vi "SIAM-StackContinous.vi"(7 "Constants":T2={"Camera-StartLine"=1, "Camera-Endline"=1024, "Trigger_ticks"=10, "zAccel"=0.05, "z-delay-ticks"=700, "SCMOS-LineSpeed [10µs]"=2.7766} {"SCMOS-LineSpeed [10µs]" format="%#.6f" items=["Fast-285MHz"=0.9175, "Slow-95MHz"=2.7525, "Slow4.2"=2.7766]}, 8 "error in (no error)":errorcluster, 11 "User":T3={"z-distance_counts"=-500, "#planes"=20, "Digital-out"=enum."Laser0", "exposue [10µs]"=9600} {"#planes" min=1}) -> (0 "error out":errorcluster, 1 "SIAMScript":T5(array[cluster])=[{"Delay 10µs"=0, "command"=3489660929, "P0"=1048576, "P1"=1048576, "P2"=0, "P3"=0, "P4"=0, "P5-ticket"=0}, {"Delay 10µs"=10, "command"=3489660929, "P0"=1, "P1"=1, "P2"=0, "P3"=0, "P4"=0, "P5-ticket"=0}, {"Delay 10µs"=0, "command"=104857633, "P0"=-213, "P1"=0, "P2"=0, "P3"=0, "P4"=0, "P5-ticket"=0}, {"Delay 10µs"=192000, "command"=3489660929, "P0"=1, "P1"=0, "P2"=0, "P3"=0, "P4"=0, "P5-ticket"=0}, {"Delay 10µs"=0, "command"=104857633, "P0"=0, "P1"=0, "P2"=0, "P3"=0, "P4"=0, "P5-ticket"=0}, {"Delay 10µs"=2840, "command"=3489660929, "P0"=1048576, "P1"=0, "P2"=0, "P3"=0, "P4"=0, "P5-ticket"=0}, {"Delay 10µs"=50, "command"=104857729, "P0"=2560000, "P1"=0, "P2"=0, "P3"=0, "P4"=0, "P5-ticket"=0}, {"Delay 10µs"=10, "command"=4027518991, "P0"=0, "P1"=0, "P2"=0, "P3"=0, "P4"=0, "P5-ticket"=112}] {"command" format="%x" items=["read_x-Motor_status_ticket"=17305600, "init_x-Motor"=17760263, "read_x-Motor_absolute_ticket"=16781312, "move_x-Motor_absolute"=16777217, "move_x-Motor_relative"=16842753, "read_x-Motor_speed"=16977920, "set_x-Motor_speed"=16973825, "read_y-Motor_status_ticket"=18354176, "init_y-Motor"=18808839, "read_y-Motor_absolute_ticket"=17829888, "move_y-Motor_absolute"=17825793, "move_y-Motor_relative"=17891329, "read_y-Motor_speed"=18026496, "set_y-Motor_speed"=18022401, "read_z-Motor_status_ticket"=19402752, "init_z-Motor"=19857415, "stop_z-Motor"=19857423, "start_z-Motor"=19857422, "read_z-Motor_absolute_ticket"=18878464, "move_z-Motor_absolute"=18874369, "move_z-Motor_relative"=18939905, "read_Objective_status_ticket"=20451328, "init_Objective"=20905991, "read_Objective_absolute_ticket"=19927040, "move_Objective_absolute"=19922945, "move_Objective_relative"=19988481, "read_Objective-Motor_speed"=20123648, "set_Objective-Motor_speed"=20119553, "read_Filter_status_ticket"=21499904, "init_Filter"=21954567, "read_Filter_absolute_ticket"=20975616, "move_Filter_absolute"=20971521, "move_Filter_relative"=21037057, "read_Filter-Motor_speed"=21172224, "set_Filter-Motor_speed"=21168129, "read_Trans-Rad_status_ticket"=22548480, "init_Trans-Rad"=23003143, "read_Trans-Rad_absolute_ticket"=22024192, "move_Trans-Rad_absolute"=22020097, "move_Trans-Rad_relative"=22085633, "read_Trans-Motor_speed"=22220800, "set_Trans-Motor_speed"=22216705, "read_FRET_status_ticket"=23597056, "init_FRET"=24051719, "read_FRET_absolute_ticket"=23072768, "move_FRET_absolute"=23068673, "move_FRET_relative"=23134209, "read_FRET-Motor_speed"=23269376, "set_FRET-Motor_speed"=23265281, "read_SI-Rad_status_ticket"=24645632, "init_SI-Rad"=25100295, "read_SI-Rad_absolute_ticket"=24121344, "move_SI-Rad_absolute"=24117249, "move_SI-Rad_relative"=24182785, "read_SI-Rad_speed"=24317952, "set_SI-Rad_speed"=24313857, "I2C-write"=335544321, "I2C-read"=335548416, "end_no_ticket"=4027514895, "end_ticket"=4027518991, "IO-read_bank0"=3489665024, "IO-write_bank0"=3489660929, "IO-read_bank1"=3506442240, "IO-write_bank1"=3506438145, "DA0-0_LED365"=2684354561, "DA0-1_LED385"=2685403137, "DA0-2_LED440"=2686451713, "DA0-3_LED470"=2687500289, "DA0-4_LED510"=2688548865, "DA0-5_LED550"=2689597441, "DA0-6_LED590"=2690646017, "DA0-7_LED640"=2691694593, "DA1-0_LED-R"=2701131777, "DA1-1_LED-G"=2702180353, "DA1-2_LED-B"=2703228929, "DA1-3_LED-AF"=2704277505, "DA1-4"=2705326081, "DA1-5"=2706374657, "DA1-6"=2707423233, "DA1-7"=2708471809, "DA2-Laser0"=2717908993, "DA2-Laser1"=2718957569, "DA2-Laser2"=2720006145, "DA2-Laser3"=2721054721, "DA2-Laser4"=2722103297, "Analog-read_AD0-0"=2818576384, "Analog-read-store_AD0-0"=2818572290, "IO-delay_bank0"=3489923073, "IO-delay_bank0_fromVar"=3489923075, "read_cam_clock"=3289124864, "store_cam_clock"=3289120770, "read_cam_phase"=3289190400, "store_cam_phase"=3289190402, "Read ticks"=4027518976, "Read ticks to var"=4027518978, "Read IP"=4043313152, "Read IP into var"=4043313154, "Set IP from var"=4043309059, "Set IP from var, relative"=4043313155, "decrement_branchRel_if_equal"=4043374945, "decrement_branchRel_if_greaterequal"=4043375201, "decrement_branchRel_if_greaterequal_withTicket"=4043379297, "decrement_branchRel_if_smaller"=4043375457, "increment_branchRel_if_smaller"=4043375473, "readVar"=4060090368, "writeVar"=4060086273, "readVar_and_copy_to_var2"=4060086275, "loadVar2_andcopy_var1"=4060086276, "math_addToVariable"=4076863488, "math_addVToVariable"=4076863489, "math_subToVariable"=4076863490, "math_subVToVariable"=4076863491, "math_multToVariable"=4076863492, "math_multvToVariable"=4076863493, "math_divideToVariable"=4076863494, "math_divideVToVariable"=4076863495, "math_modToVariable"=4076863496, "math_modVToVariable"=4076863497, "logic_and"=4093640704, "logic_or"=4093640706, "logic_xor"=4093640708, "set_1Galvo"=101712113, "set_x-Galvo"=102760689, "set_y-Galvo"=103809265, "set_z-Fokus"=104857841, "set_1Galvo_position-only"=101711937, "set_x-Galvo_position-only"=102760513, "set_y-Galvo_position-only"=103809089, "set_z-Fokus_position-only"=104857665, "set_x-Galvo_position-only_ticket"=102764609, "set_y-Galvo_position-only_ticket"=103813185, "set_z-Fokus_position-only_ticket"=104861761, "set_x-Galvo_relativ-only"=102760577, "set_y-Galvo_relativ-only"=103809153, "set_z-Fokus_relativ-only"=104857729, "set_x-Galvo_speed-only"=102760481, "set_y-Galvo_speed-only"=103809057, "set_z-Fokus_speed-only"=104857633, "read_1Galvo_ticket"=101716032, "read_x-Galvo_ticket"=102764608, "read_y-Galvo_ticket"=103813184, "read_z-Focus_ticket"=104861760, "x-Galvo_pos_fromVar"=102760515, "y-Galvo_pos_fromVar"=103809091, "z-Focus_pos_fromVar"=104857667, "Servo0"=67108865, "Servo0-enable"=68091911, "Servo0-disable"=68091919, "Servo1"=68157441, "Servo1-enable"=69140487, "Servo1-disable"=69140495, "EnablePower0-SM"=2148466695, "DisablePower0-SM"=2148466703, "EnablePower1-Thermo1"=2149515271, "DisablePower1-Thermo1"=2149515279, "EnablePower2-Cam"=2150563847, "DisablePower2-Cam"=2150563855, "EnablePower3-Thermo2"=2151612423, "DisablePower3-Thermo2"=2151612431, "EnablePower4-Laser0"=2152660999, "DisablePower4-Laser0"=2152661007, "EnablePower5"=2153709575, "DisablePower5"=2153709583, "EnablePower6-Laser1"=2154758151, "DisablePower6-Laser1"=2154758159, "EnablePower7-SAM"=2155806727, "DisablePower7-SAM"=2155806735, "EnablePower8-Laser2"=2156855303, "DisablePower8-Laser2"=2156855311, "EnablePower9-TSM"=2157903879, "DisablePower9-TSM"=2157903887, "EnablePower10-Laser3"=2158952455, "DisablePower10-Laser3"=2158952463, "EnablePower11-Servo"=2160001031, "DisablePower11-Servo"=2160001039, "EnablePower12-Laser4"=2161049607, "DisablePower12-Laser4"=2161049615, "EnableSMPower2-DCC22"=2167341063, "DisableSMPower2-DCC22"=2167341071, "EnableSMPower3-6220"=2168389639, "DisableSMPower3-6220"=2168389647, "EnableSMPower4-6210"=2169438215, "DisableSMPower4-6210"=2169438223]}, 2 "Camera":T1={"Camera-Exposure µs"=96000.0, "CameraImages"=20})   [LabVIEW 2011]
uses:
  SIAM_command.ctl
panel:
  out "readout":u32=2840
  out "size(s)":i32=8
  # "1.laser an\n2. trigger an\n3. linaer z bewegen, linear geht naicht also lauter schritte\n4. trigger aus\n5. laser aus\n6. z stop, Readout später!\n7. z zurück\n8 ende\nCamware macht sequenz!"
  # "var0=phase\nvar1=clock256\nvar 2 =linecounter \nvar 3 =framecounter"
  # "<-- user inputs --------------------------- constants ---->"
  # "-250 count = 500nm"
  # "Pixel definition: 0\nmiddel: lines\nbottom +2lines"
  # "alles umstellen auf count und Pixel und 10µs !!!"
  # "lineclock read slow=AD99E =711070 =/256=27.77617"
  # "a gerechnet wobbler~3.7, x~98, eher /2\nz~6ms/2µm"
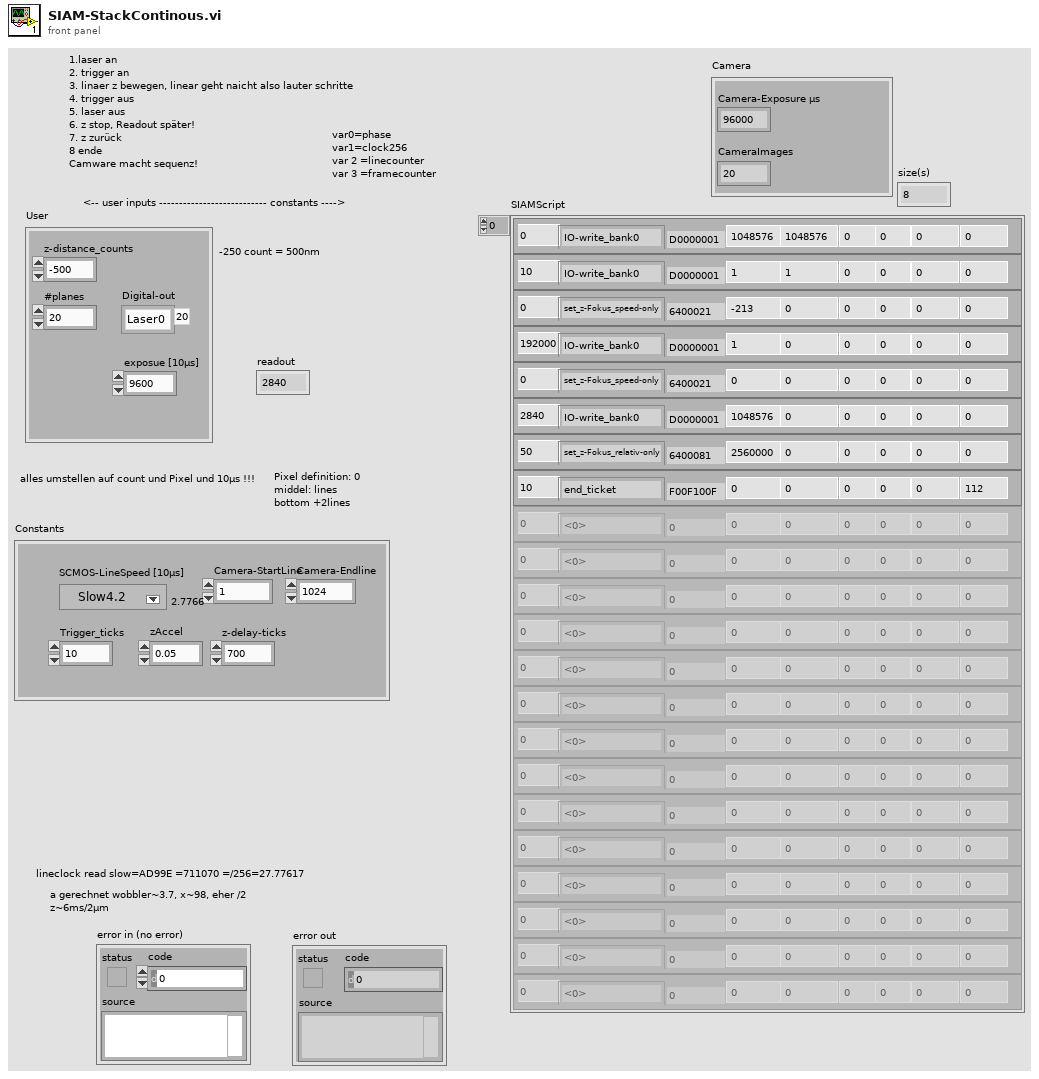
[diagram p1: front panel]
types:
  T1 = cluster{"Camera-Exposure µs":dbl, "CameraImages":u16}
  T2 = cluster{"Camera-StartLine":u32, "Camera-Endline":u32, "Trigger_ticks":u32, "zAccel":dbl, "z-delay-ticks":u32, "SCMOS-LineSpeed [10µs]":dbl}
  T3 = cluster{"z-distance_counts":i32, "#planes":u16, "Digital-out":enum8{"cam1", "cam1-ready?", "cam2", "cam2-ready?", "tmsx?", "tsmy?", "tsm3?", "lid?", "led1", "led2", "led3", "led4", "led5", "led6", "led7", "led8", "durchR", "durchG", "durchB", "AF", "Laser0", "Laser1", "Laser2", "Laser3", "Laser4", "LaserX", "TrigOut", "SMB1", ""}, "exposue [10µs]":u32}
  T4 = typedef "SIAM_command.ctl" = u32
  T5 = cluster{"Delay 10µs":u32, "command":T4, "P0":i32, "P1":i32, "P2":i32, "P3":i32, "P4":i32, "P5-ticket":i32}[]
  T6 = cluster{"Delay 10µs":u32, "command":T4, "P0":i32, "P1":i32, "P2":i32, "P3":i32, "P4":i32, "P5-ticket":i32}
  T7 = cluster{"Camera-Exposure":dbl, "CameraImages":u16}
  T8 = enum8{"Ch0", "Ch1", "x-Galvo", "y-Galvo", "z-Focus"}
  T9 = enum8{"cam1", "cam1-ready?", "cam2", "cam2-ready?", "tmsx?", "tsmy?", "tsm3?", "lid?", "led1", "led2", "led3", "led4", "led5", "led6", "led7", "led8", "durchR", "durchG", "durchB", "AF", "Laser0", "Laser1", "Laser2", "Laser3", "Laser4", "LaserX", "TrigOut", "SMB1", ""}
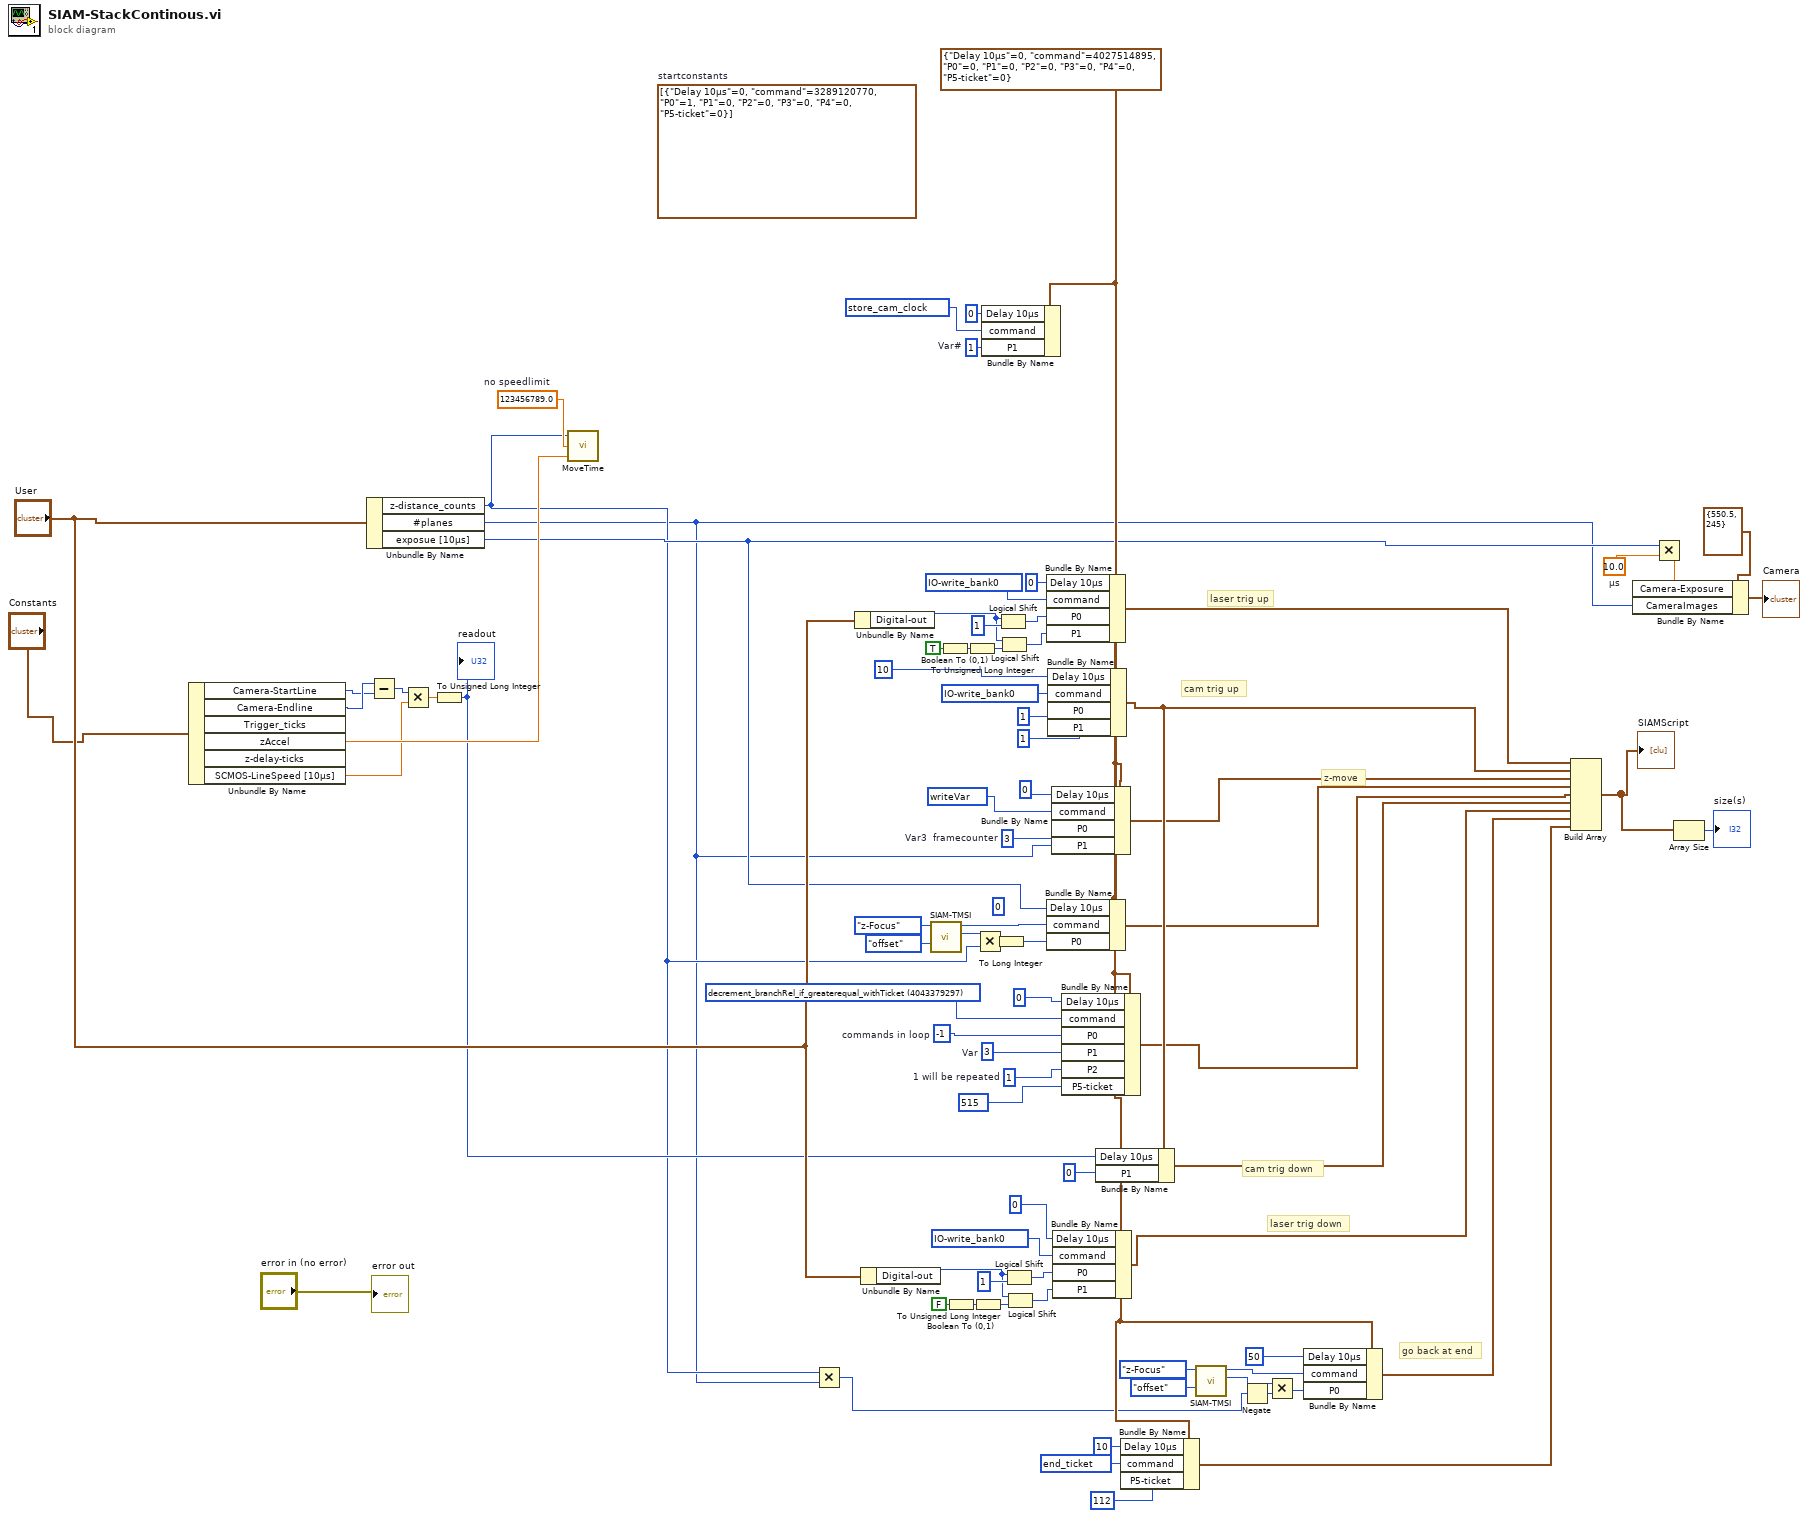
[diagram p0: block diagram]
diagram:
  w11 = 1  # 1 will be repeated
  w13 = 3  # Var
  w10 = -1  # commands in loop
  w14 = T4 4043379297 items=["read_x-Motor_status_ticket"=17305600, "init_x-Motor"=17760263, "read_x-Motor_absolute_ticket"=16781312, "move_x-Motor_absolute"=16777217, "move_x-Motor_relative"=16842753, "read_x-Motor_speed"=16977920, "set_x-Motor_speed"=16973825, "read_y-Motor_status_ticket"=18354176, "init_y-Motor"=18808839, "read_y-Motor_absolute_ticket"=17829888, "move_y-Motor_absolute"=17825793, "move_y-Motor_relative"=17891329, "read_y-Motor_speed"=18026496, "set_y-Motor_speed"=18022401, "read_z-Motor_status_ticket"=19402752, "init_z-Motor"=19857415, "stop_z-Motor"=19857423, "start_z-Motor"=19857422, "read_z-Motor_absolute_ticket"=18878464, "move_z-Motor_absolute"=18874369, "move_z-Motor_relative"=18939905, "read_Objective_status_ticket"=20451328, "init_Objective"=20905991, "read_Objective_absolute_ticket"=19927040, "move_Objective_absolute"=19922945, "move_Objective_relative"=19988481, "read_Objective-Motor_speed"=20123648, "set_Objective-Motor_speed"=20119553, "read_Filter_status_ticket"=21499904, "init_Filter"=21954567, "read_Filter_absolute_ticket"=20975616, "move_Filter_absolute"=20971521, "move_Filter_relative"=21037057, "read_Filter-Motor_speed"=21172224, "set_Filter-Motor_speed"=21168129, "read_Trans-Rad_status_ticket"=22548480, "init_Trans-Rad"=23003143, "read_Trans-Rad_absolute_ticket"=22024192, "move_Trans-Rad_absolute"=22020097, "move_Trans-Rad_relative"=22085633, "read_Trans-Motor_speed"=22220800, "set_Trans-Motor_speed"=22216705, "read_FRET_status_ticket"=23597056, "init_FRET"=24051719, "read_FRET_absolute_ticket"=23072768, "move_FRET_absolute"=23068673, "move_FRET_relative"=23134209, "read_FRET-Motor_speed"=23269376, "set_FRET-Motor_speed"=23265281, "read_SI-Rad_status_ticket"=24645632, "init_SI-Rad"=25100295, "read_SI-Rad_absolute_ticket"=24121344, "move_SI-Rad_absolute"=24117249, "move_SI-Rad_relative"=24182785, "read_SI-Rad_speed"=24317952, "set_SI-Rad_speed"=24313857, "end_no_ticket"=4027514895, "end_ticket"=4027518991, "IO-read_bank0"=3489665024, "IO-write_bank0"=3489660929, "IO-read_bank1"=3506442240, "IO-write_bank1"=3506438145, "DA0-0_LED365"=2684354561, "DA0-1_LED385"=2685403137, "DA0-2_LED440"=2686451713, "DA0-3_LED470"=2687500289, "DA0-4_LED510"=2688548865, "DA0-5_LED550"=2689597441, "DA0-6_LED590"=2690646017, "DA0-7_LED640"=2691694593, "DA1-0_LED-R"=2701131777, "DA1-1_LED-G"=2702180353, "DA1-2_LED-B"=2703228929, "DA1-3_LED-AF"=2704277505, "DA1-4"=2705326081, "DA1-5"=2706374657, "DA1-6"=2707423233, "DA1-7"=2708471809, "DA2-Laser0"=2717908993, "DA2-Laser1"=2718957569, "DA2-Laser2"=2720006145, "DA2-Laser3"=2721054721, "DA2-Laser4"=2722103297, "Analog-read_AD0-0"=2818576384, "Analog-read-store_AD0-0"=2818572290, "IO-delay_bank0"=3489923073, "IO-delay_bank0_fromVar"=3489923075, "read_cam_clock"=3289124864, "store_cam_clock"=3289120770, "read_cam_phase"=3289190400, "store_cam_phase"=3289190402, "Read ticks"=4027518976, "Read ticks to var"=4027518978, "Read IP"=4043313152, "Read IP into var"=4043313154, "Set IP from var"=4043309059, "Set IP from var, relative"=4043313155, "decrement_branchRel_if_equal"=4043374945, "decrement_branchRel_if_greaterequal"=4043375201, "decrement_branchRel_if_greaterequal_withTicket"=4043379297, "decrement_branchRel_if_smaller"=4043375457, "increment_branchRel_if_smaller"=4043375473, "readVar"=4060090368, "writeVar"=4060086273, "readVar_and_copy_to_var2"=4060086275, "loadVar2_andcopy_var1"=4060086276, "math_addToVariable"=4076863488, "math_addVToVariable"=4076863489, "math_subToVariable"=4076863490, "math_subVToVariable"=4076863491, "math_multToVariable"=4076863492, "math_multvToVariable"=4076863493, "math_divideToVariable"=4076863494, "math_divideVToVariable"=4076863495, "math_modToVariable"=4076863496, "math_modVToVariable"=4076863497, "logic_and"=4093640704, "logic_or"=4093640706, "logic_xor"=4093640708, "set_1Galvo"=101712113, "set_x-Galvo"=102760689, "set_y-Galvo"=103809265, "set_z-Fokus"=104857841, "set_1Galvo_position-only"=101711937, "set_x-Galvo_position-only"=102760513, "set_y-Galvo_position-only"=103809089, "set_z-Fokus_position-only"=104857665, "set_x-Galvo_position-only_ticket"=102764609, "set_y-Galvo_position-only_ticket"=103813185, "set_z-Fokus_position-only_ticket"=104861761, "set_x-Galvo_relativ-only"=102760577, "set_y-Galvo_relativ-only"=103809153, "set_z-Fokus_relativ-only"=104857729, "set_x-Galvo_speed-only"=102760481, "set_y-Galvo_speed-only"=103809057, "set_z-Fokus_speed-only"=104857633, "read_1Galvo_ticket"=101716032, "read_x-Galvo_ticket"=102764608, "read_y-Galvo_ticket"=103813184, "read_z-Focus_ticket"=104861760, "x-Galvo_pos_fromVar"=102760515, "y-Galvo_pos_fromVar"=103809091, "z-Focus_pos_fromVar"=104857667, "Servo0"=67108865, "Servo0-enable"=68091911, "Servo0-disable"=68091919, "Servo1"=68157441, "Servo1-enable"=69140487, "Servo1-disable"=69140495, "EnablePower0-SM"=2148466695, "DisablePower0-SM"=2148466703, "EnablePower1-Thermo1"=2149515271, "DisablePower1-Thermo1"=2149515279, "EnablePower2-Cam"=2150563847, "DisablePower2-Cam"=2150563855, "EnablePower3-Thermo2"=2151612423, "DisablePower3-Thermo2"=2151612431, "EnablePower4-Laser0"=2152660999, "DisablePower4-Laser0"=2152661007, "EnablePower5"=2153709575, "DisablePower5"=2153709583, "EnablePower6-Laser1"=2154758151, "DisablePower6-Laser1"=2154758159, "EnablePower7-SAM"=2155806727, "DisablePower7-SAM"=2155806735, "EnablePower8-Laser2"=2156855303, "DisablePower8-Laser2"=2156855311, "EnablePower9-TSM"=2157903879, "DisablePower9-TSM"=2157903887, "EnablePower10-Laser3"=2158952455, "DisablePower10-Laser3"=2158952463, "EnablePower11-Servo"=2160001031, "DisablePower11-Servo"=2160001039, "EnablePower12-Laser4"=2161049607, "DisablePower12-Laser4"=2161049615, "EnableSMPower2-DCC22"=2167341063, "DisableSMPower2-DCC22"=2167341071, "EnableSMPower3-6220"=2168389639, "DisableSMPower3-6220"=2168389647, "EnableSMPower4-6210"=2169438215, "DisableSMPower4-6210"=2169438223] ("command")
  w15 = 3  # Var3  framecounter
  w17 = T4 4060086273 items=["read_x-Motor_status_ticket"=17305600, "init_x-Motor"=17760263, "read_x-Motor_absolute_ticket"=16781312, "move_x-Motor_absolute"=16777217, "move_x-Motor_relative"=16842753, "read_x-Motor_speed"=16977920, "set_x-Motor_speed"=16973825, "read_y-Motor_status_ticket"=18354176, "init_y-Motor"=18808839, "read_y-Motor_absolute_ticket"=17829888, "move_y-Motor_absolute"=17825793, "move_y-Motor_relative"=17891329, "read_y-Motor_speed"=18026496, "set_y-Motor_speed"=18022401, "read_z-Motor_status_ticket"=19402752, "init_z-Motor"=19857415, "stop_z-Motor"=19857423, "start_z-Motor"=19857422, "read_z-Motor_absolute_ticket"=18878464, "move_z-Motor_absolute"=18874369, "move_z-Motor_relative"=18939905, "read_Objective_status_ticket"=20451328, "init_Objective"=20905991, "read_Objective_absolute_ticket"=19927040, "move_Objective_absolute"=19922945, "move_Objective_relative"=19988481, "read_Objective-Motor_speed"=20123648, "set_Objective-Motor_speed"=20119553, "read_Filter_status_ticket"=21499904, "init_Filter"=21954567, "read_Filter_absolute_ticket"=20975616, "move_Filter_absolute"=20971521, "move_Filter_relative"=21037057, "read_Filter-Motor_speed"=21172224, "set_Filter-Motor_speed"=21168129, "read_Trans-Rad_status_ticket"=22548480, "init_Trans-Rad"=23003143, "read_Trans-Rad_absolute_ticket"=22024192, "move_Trans-Rad_absolute"=22020097, "move_Trans-Rad_relative"=22085633, "read_Trans-Motor_speed"=22220800, "set_Trans-Motor_speed"=22216705, "read_FRET_status_ticket"=23597056, "init_FRET"=24051719, "read_FRET_absolute_ticket"=23072768, "move_FRET_absolute"=23068673, "move_FRET_relative"=23134209, "read_FRET-Motor_speed"=23269376, "set_FRET-Motor_speed"=23265281, "read_SI-Rad_status_ticket"=24645632, "init_SI-Rad"=25100295, "read_SI-Rad_absolute_ticket"=24121344, "move_SI-Rad_absolute"=24117249, "move_SI-Rad_relative"=24182785, "read_SI-Rad_speed"=24317952, "set_SI-Rad_speed"=24313857, "end_no_ticket"=4027514895, "end_ticket"=4027518991, "IO-read_bank0"=3489665024, "IO-write_bank0"=3489660929, "IO-read_bank1"=3506442240, "IO-write_bank1"=3506438145, "DA0-0_LED365"=2684354561, "DA0-1_LED385"=2685403137, "DA0-2_LED440"=2686451713, "DA0-3_LED470"=2687500289, "DA0-4_LED510"=2688548865, "DA0-5_LED550"=2689597441, "DA0-6_LED590"=2690646017, "DA0-7_LED640"=2691694593, "DA1-0_LED-R"=2701131777, "DA1-1_LED-G"=2702180353, "DA1-2_LED-B"=2703228929, "DA1-3_LED-AF"=2704277505, "DA1-4"=2705326081, "DA1-5"=2706374657, "DA1-6"=2707423233, "DA1-7"=2708471809, "DA2-Laser0"=2717908993, "DA2-Laser1"=2718957569, "DA2-Laser2"=2720006145, "DA2-Laser3"=2721054721, "DA2-Laser4"=2722103297, "Analog-read_AD0-0"=2818576384, "Analog-read-store_AD0-0"=2818572290, "IO-delay_bank0"=3489923073, "IO-delay_bank0_fromVar"=3489923075, "read_cam_clock"=3289124864, "store_cam_clock"=3289120770, "read_cam_phase"=3289190400, "store_cam_phase"=3289190402, "Read ticks"=4027518976, "Read ticks to var"=4027518978, "Read IP"=4043313152, "Read IP into var"=4043313154, "Set IP from var"=4043309059, "Set IP from var, relative"=4043313155, "decrement_branchRel_if_equal"=4043374945, "decrement_branchRel_if_greaterequal"=4043375201, "decrement_branchRel_if_greaterequal_withTicket"=4043379297, "decrement_branchRel_if_smaller"=4043375457, "increment_branchRel_if_smaller"=4043375473, "readVar"=4060090368, "writeVar"=4060086273, "readVar_and_copy_to_var2"=4060086275, "loadVar2_andcopy_var1"=4060086276, "math_addToVariable"=4076863488, "math_addVToVariable"=4076863489, "math_subToVariable"=4076863490, "math_subVToVariable"=4076863491, "math_multToVariable"=4076863492, "math_multvToVariable"=4076863493, "math_divideToVariable"=4076863494, "math_divideVToVariable"=4076863495, "math_modToVariable"=4076863496, "math_modVToVariable"=4076863497, "logic_and"=4093640704, "logic_or"=4093640706, "logic_xor"=4093640708, "set_1Galvo"=101712113, "set_x-Galvo"=102760689, "set_y-Galvo"=103809265, "set_z-Fokus"=104857841, "set_1Galvo_position-only"=101711937, "set_x-Galvo_position-only"=102760513, "set_y-Galvo_position-only"=103809089, "set_z-Fokus_position-only"=104857665, "set_x-Galvo_position-only_ticket"=102764609, "set_y-Galvo_position-only_ticket"=103813185, "set_z-Fokus_position-only_ticket"=104861761, "set_x-Galvo_relativ-only"=102760577, "set_y-Galvo_relativ-only"=103809153, "set_z-Fokus_relativ-only"=104857729, "set_x-Galvo_speed-only"=102760481, "set_y-Galvo_speed-only"=103809057, "set_z-Fokus_speed-only"=104857633, "read_1Galvo_ticket"=101716032, "read_x-Galvo_ticket"=102764608, "read_y-Galvo_ticket"=103813184, "read_z-Focus_ticket"=104861760, "x-Galvo_pos_fromVar"=102760515, "y-Galvo_pos_fromVar"=103809091, "z-Focus_pos_fromVar"=104857667, "Servo0"=67108865, "Servo0-enable"=68091911, "Servo0-disable"=68091919, "Servo1"=68157441, "Servo1-enable"=69140487, "Servo1-disable"=69140495, "EnablePower0-SM"=2148466695, "DisablePower0-SM"=2148466703, "EnablePower1-Thermo1"=2149515271, "DisablePower1-Thermo1"=2149515279, "EnablePower2-Cam"=2150563847, "DisablePower2-Cam"=2150563855, "EnablePower3-Thermo2"=2151612423, "DisablePower3-Thermo2"=2151612431, "EnablePower4-Laser0"=2152660999, "DisablePower4-Laser0"=2152661007, "EnablePower5"=2153709575, "DisablePower5"=2153709583, "EnablePower6-Laser1"=2154758151, "DisablePower6-Laser1"=2154758159, "EnablePower7-SAM"=2155806727, "DisablePower7-SAM"=2155806735, "EnablePower8-Laser2"=2156855303, "DisablePower8-Laser2"=2156855311, "EnablePower9-TSM"=2157903879, "DisablePower9-TSM"=2157903887, "EnablePower10-Laser3"=2158952455, "DisablePower10-Laser3"=2158952463, "EnablePower11-Servo"=2160001031, "DisablePower11-Servo"=2160001039, "EnablePower12-Laser4"=2161049607, "DisablePower12-Laser4"=2161049615, "EnableSMPower2-DCC22"=2167341063, "DisableSMPower2-DCC22"=2167341071, "EnableSMPower3-6220"=2168389639, "DisableSMPower3-6220"=2168389647, "EnableSMPower4-6210"=2169438215, "DisableSMPower4-6210"=2169438223] ("command")
  w35 = 123456789.0  # no speedlimit
  w44 = T4 3489660929 items=["read_x-Motor_status_ticket"=17305600, "init_x-Motor"=17760263, "read_x-Motor_absolute_ticket"=16781312, "move_x-Motor_absolute"=16777217, "move_x-Motor_relative"=16842753, "read_y-Motor_status_ticket"=18354176, "init_y-Motor"=18808839, "read_y-Motor_absolute_ticket"=17829888, "move_y-Motor_absolute"=17825793, "move_y-Motor_relative"=17891329, "read_z-Motor_status_ticket"=19402752, "init_z-Motor"=19857415, "stop_z-Motor"=19857423, "start_z-Motor"=19857422, "read_z-Motor_absolute_ticket"=18878464, "move_z-Motor_absolute"=18874369, "move_z-Motor_relative"=18939905, "end_no_ticket"=4027514895, "end_ticket"=4027518991, "IO-read_bank0"=3489665024, "IO-write_bank0"=3489660929, "IO-read_bank1"=3506442240, "IO-write_bank1"=3506438145, "IO-delay_bank0"=3489923073, "IO-delay_bank0_fromVar"=3489923075, "read_cam_clock"=3289124864, "store_cam_clock"=3289120770, "read_cam_phase"=3289190400, "set_cam_deadtime"=3288989697, "set_cam_10uscycles"=3289055233, "set_cam_10uscycles_fromVariable"=3289055235, "calc_cam"=3289317386, "store_cam_Var"=3289251842, "math_addToVariable"=4060086278, "readVar"=4060090368, "writeVar"=4060086273, "copyVar"=4060086276, "decrement_branchRel_if_equal"=4043374945, "decrement_branchRel_if_greaterequal"=4043375201, "decrement_branchRel_if_greaterequal_withTicket"=4043379297, "decrement_branchRel_if_smaller"=4043375457, "increment_branchRel_if_smaller"=4043375473, "set_x-Galvo"=1612710129, "set_y-Galvo"=1613758705, "set_z-Fokus"=1614807281, "set_x-Galvo_position-only"=1612709953, "set_y-Galvo_position-only"=1613758529, "set_z-Fokus_position-only"=1614807105, "set_x-Galvo_position-only_ticket"=1612714049, "set_y-Galvo_position-only_ticket"=1613762625, "set_z-Fokus_position-only_ticket"=1614811201, "read_x-Galvo_ticket"=1612714048, "read_y-Galvo_ticket"=1613762624, "read_z-Focus_ticket"=1614811200, "x-Galvo_pos_fromVar"=1612709955, "y-Galvo_pos_fromVar"=1613758531, "z-Focus_pos_fromVar"=1614807107] ("command")
  w52 = T4 3489660929 items=["read_x-Motor_status_ticket"=17305600, "init_x-Motor"=17760263, "read_x-Motor_absolute_ticket"=16781312, "move_x-Motor_absolute"=16777217, "move_x-Motor_relative"=16842753, "read_y-Motor_status_ticket"=18354176, "init_y-Motor"=18808839, "read_y-Motor_absolute_ticket"=17829888, "move_y-Motor_absolute"=17825793, "move_y-Motor_relative"=17891329, "read_z-Motor_status_ticket"=19402752, "init_z-Motor"=19857415, "stop_z-Motor"=19857423, "start_z-Motor"=19857422, "read_z-Motor_absolute_ticket"=18878464, "move_z-Motor_absolute"=18874369, "move_z-Motor_relative"=18939905, "end_no_ticket"=4027514895, "end_ticket"=4027518991, "IO-read_bank0"=3489665024, "IO-write_bank0"=3489660929, "IO-read_bank1"=3506442240, "IO-write_bank1"=3506438145, "IO-delay_bank0"=3489923073, "IO-delay_bank0_fromVar"=3489923075, "read_cam_clock"=3289124864, "store_cam_clock"=3289120770, "read_cam_phase"=3289190400, "set_cam_deadtime"=3288989697, "set_cam_10uscycles"=3289055233, "set_cam_10uscycles_fromVariable"=3289055235, "calc_cam"=3289317386, "store_cam_Var"=3289251842, "math_addToVariable"=4060086278, "readVar"=4060090368, "writeVar"=4060086273, "copyVar"=4060086276, "decrement_branchRel_if_equal"=4043374945, "decrement_branchRel_if_greaterequal"=4043375201, "decrement_branchRel_if_greaterequal_withTicket"=4043379297, "decrement_branchRel_if_smaller"=4043375457, "increment_branchRel_if_smaller"=4043375473, "set_x-Galvo"=1612710129, "set_y-Galvo"=1613758705, "set_z-Fokus"=1614807281, "set_x-Galvo_position-only"=1612709953, "set_y-Galvo_position-only"=1613758529, "set_z-Fokus_position-only"=1614807105, "set_x-Galvo_position-only_ticket"=1612714049, "set_y-Galvo_position-only_ticket"=1613762625, "set_z-Fokus_position-only_ticket"=1614811201, "read_x-Galvo_ticket"=1612714048, "read_y-Galvo_ticket"=1613762624, "read_z-Focus_ticket"=1614811200, "x-Galvo_pos_fromVar"=1612709955, "y-Galvo_pos_fromVar"=1613758531, "z-Focus_pos_fromVar"=1614807107] ("command")
  w9 = T6 {"Delay 10µs"=0, "command"=4027514895, "P0"=0, "P1"=0, "P2"=0, "P3"=0, "P4"=0, "P5-ticket"=0} ("Cluster")
  (unwired) T5 [{"Delay 10µs"=0, "command"=3289120770, "P0"=1, "P1"=0, "P2"=0, "P3"=0, "P4"=0, "P5-ticket"=0}]  # startconstants
  w53 = 1  # Var#
  w54 = T4 3289120770 items=["read_x-Motor_status_ticket"=17305600, "init_x-Motor"=17760263, "read_x-Motor_absolute_ticket"=16781312, "move_x-Motor_absolute"=16777217, "move_x-Motor_relative"=16842753, "read_x-Motor_speed"=16977920, "set_x-Motor_speed"=16973825, "read_y-Motor_status_ticket"=18354176, "init_y-Motor"=18808839, "read_y-Motor_absolute_ticket"=17829888, "move_y-Motor_absolute"=17825793, "move_y-Motor_relative"=17891329, "read_y-Motor_speed"=18026496, "set_y-Motor_speed"=18022401, "read_z-Motor_status_ticket"=19402752, "init_z-Motor"=19857415, "stop_z-Motor"=19857423, "start_z-Motor"=19857422, "read_z-Motor_absolute_ticket"=18878464, "move_z-Motor_absolute"=18874369, "move_z-Motor_relative"=18939905, "read_Objective_status_ticket"=20451328, "init_Objective"=20905991, "read_Objective_absolute_ticket"=19927040, "move_Objective_absolute"=19922945, "move_Objective_relative"=19988481, "read_Objective-Motor_speed"=20123648, "set_Objective-Motor_speed"=20119553, "read_Filter_status_ticket"=21499904, "init_Filter"=21954567, "read_Filter_absolute_ticket"=20975616, "move_Filter_absolute"=20971521, "move_Filter_relative"=21037057, "read_Filter-Motor_speed"=21172224, "set_Filter-Motor_speed"=21168129, "read_Trans-Rad_status_ticket"=22548480, "init_Trans-Rad"=23003143, "read_Trans-Rad_absolute_ticket"=22024192, "move_Trans-Rad_absolute"=22020097, "move_Trans-Rad_relative"=22085633, "read_Trans-Motor_speed"=22220800, "set_Trans-Motor_speed"=22216705, "read_FRET_status_ticket"=23597056, "init_FRET"=24051719, "read_FRET_absolute_ticket"=23072768, "move_FRET_absolute"=23068673, "move_FRET_relative"=23134209, "read_FRET-Motor_speed"=23269376, "set_FRET-Motor_speed"=23265281, "read_SI-Rad_status_ticket"=24645632, "init_SI-Rad"=25100295, "read_SI-Rad_absolute_ticket"=24121344, "move_SI-Rad_absolute"=24117249, "move_SI-Rad_relative"=24182785, "read_SI-Rad_speed"=24317952, "set_SI-Rad_speed"=24313857, "I2C-write"=335544321, "I2C-read"=335548416, "end_no_ticket"=4027514895, "end_ticket"=4027518991, "IO-read_bank0"=3489665024, "IO-write_bank0"=3489660929, "IO-read_bank1"=3506442240, "IO-write_bank1"=3506438145, "DA0-0_LED365"=2684354561, "DA0-1_LED385"=2685403137, "DA0-2_LED440"=2686451713, "DA0-3_LED470"=2687500289, "DA0-4_LED510"=2688548865, "DA0-5_LED550"=2689597441, "DA0-6_LED590"=2690646017, "DA0-7_LED640"=2691694593, "DA1-0_LED-R"=2701131777, "DA1-1_LED-G"=2702180353, "DA1-2_LED-B"=2703228929, "DA1-3_LED-AF"=2704277505, "DA1-4"=2705326081, "DA1-5"=2706374657, "DA1-6"=2707423233, "DA1-7"=2708471809, "DA2-Laser0"=2717908993, "DA2-Laser1"=2718957569, "DA2-Laser2"=2720006145, "DA2-Laser3"=2721054721, "DA2-Laser4"=2722103297, "Analog-read_AD0-0"=2818576384, "Analog-read-store_AD0-0"=2818572290, "IO-delay_bank0"=3489923073, "IO-delay_bank0_fromVar"=3489923075, "read_cam_clock"=3289124864, "store_cam_clock"=3289120770, "read_cam_phase"=3289190400, "store_cam_phase"=3289190402, "Read ticks"=4027518976, "Read ticks to var"=4027518978, "Read IP"=4043313152, "Read IP into var"=4043313154, "Set IP from var"=4043309059, "Set IP from var, relative"=4043313155, "decrement_branchRel_if_equal"=4043374945, "decrement_branchRel_if_greaterequal"=4043375201, "decrement_branchRel_if_greaterequal_withTicket"=4043379297, "decrement_branchRel_if_smaller"=4043375457, "increment_branchRel_if_smaller"=4043375473, "readVar"=4060090368, "writeVar"=4060086273, "readVar_and_copy_to_var2"=4060086275, "loadVar2_andcopy_var1"=4060086276, "math_addToVariable"=4076863488, "math_addVToVariable"=4076863489, "math_subToVariable"=4076863490, "math_subVToVariable"=4076863491, "math_multToVariable"=4076863492, "math_multvToVariable"=4076863493, "math_divideToVariable"=4076863494, "math_divideVToVariable"=4076863495, "math_modToVariable"=4076863496, "math_modVToVariable"=4076863497, "logic_and"=4093640704, "logic_or"=4093640706, "logic_xor"=4093640708, "set_1Galvo"=101712113, "set_x-Galvo"=102760689, "set_y-Galvo"=103809265, "set_z-Fokus"=104857841, "set_1Galvo_position-only"=101711937, "set_x-Galvo_position-only"=102760513, "set_y-Galvo_position-only"=103809089, "set_z-Fokus_position-only"=104857665, "set_x-Galvo_position-only_ticket"=102764609, "set_y-Galvo_position-only_ticket"=103813185, "set_z-Fokus_position-only_ticket"=104861761, "set_x-Galvo_relativ-only"=102760577, "set_y-Galvo_relativ-only"=103809153, "set_z-Fokus_relativ-only"=104857729, "set_x-Galvo_speed-only"=102760481, "set_y-Galvo_speed-only"=103809057, "set_z-Fokus_speed-only"=104857633, "read_1Galvo_ticket"=101716032, "read_x-Galvo_ticket"=102764608, "read_y-Galvo_ticket"=103813184, "read_z-Focus_ticket"=104861760, "x-Galvo_pos_fromVar"=102760515, "y-Galvo_pos_fromVar"=103809091, "z-Focus_pos_fromVar"=104857667, "Servo0"=67108865, "Servo0-enable"=68091911, "Servo0-disable"=68091919, "Servo1"=68157441, "Servo1-enable"=69140487, "Servo1-disable"=69140495, "EnablePower0-SM"=2148466695, "DisablePower0-SM"=2148466703, "EnablePower1-Thermo1"=2149515271, "DisablePower1-Thermo1"=2149515279, "EnablePower2-Cam"=2150563847, "DisablePower2-Cam"=2150563855, "EnablePower3-Thermo2"=2151612423, "DisablePower3-Thermo2"=2151612431, "EnablePower4-Laser0"=2152660999, "DisablePower4-Laser0"=2152661007, "EnablePower5"=2153709575, "DisablePower5"=2153709583, "EnablePower6-Laser1"=2154758151, "DisablePower6-Laser1"=2154758159, "EnablePower7-SAM"=2155806727, "DisablePower7-SAM"=2155806735, "EnablePower8-Laser2"=2156855303, "DisablePower8-Laser2"=2156855311, "EnablePower9-TSM"=2157903879, "DisablePower9-TSM"=2157903887, "EnablePower10-Laser3"=2158952455, "DisablePower10-Laser3"=2158952463, "EnablePower11-Servo"=2160001031, "DisablePower11-Servo"=2160001039, "EnablePower12-Laser4"=2161049607, "DisablePower12-Laser4"=2161049615, "EnableSMPower2-DCC22"=2167341063, "DisableSMPower2-DCC22"=2167341071, "EnableSMPower3-6220"=2168389639, "DisableSMPower3-6220"=2168389647, "EnableSMPower4-6210"=2169438215, "DisableSMPower4-6210"=2169438223] ("command")
  w59 = T4 3489660929 items=["read_x-Motor_status_ticket"=17305600, "init_x-Motor"=17760263, "read_x-Motor_absolute_ticket"=16781312, "move_x-Motor_absolute"=16777217, "move_x-Motor_relative"=16842753, "read_y-Motor_status_ticket"=18354176, "init_y-Motor"=18808839, "read_y-Motor_absolute_ticket"=17829888, "move_y-Motor_absolute"=17825793, "move_y-Motor_relative"=17891329, "read_z-Motor_status_ticket"=19402752, "init_z-Motor"=19857415, "stop_z-Motor"=19857423, "start_z-Motor"=19857422, "read_z-Motor_absolute_ticket"=18878464, "move_z-Motor_absolute"=18874369, "move_z-Motor_relative"=18939905, "end_no_ticket"=4027514895, "end_ticket"=4027518991, "IO-read_bank0"=3489665024, "IO-write_bank0"=3489660929, "IO-read_bank1"=3506442240, "IO-write_bank1"=3506438145, "IO-delay_bank0"=3489923073, "IO-delay_bank0_fromVar"=3489923075, "read_cam_clock"=3289124864, "store_cam_clock"=3289120770, "read_cam_phase"=3289190400, "set_cam_deadtime"=3288989697, "set_cam_10uscycles"=3289055233, "set_cam_10uscycles_fromVariable"=3289055235, "calc_cam"=3289317386, "store_cam_Var"=3289251842, "math_addToVariable"=4060086278, "readVar"=4060090368, "writeVar"=4060086273, "copyVar"=4060086276, "decrement_branchRel_if_equal"=4043374945, "decrement_branchRel_if_greaterequal"=4043375201, "decrement_branchRel_if_greaterequal_withTicket"=4043379297, "decrement_branchRel_if_smaller"=4043375457, "increment_branchRel_if_smaller"=4043375473, "set_x-Galvo"=1612710129, "set_y-Galvo"=1613758705, "set_z-Fokus"=1614807281, "set_x-Galvo_position-only"=1612709953, "set_y-Galvo_position-only"=1613758529, "set_z-Fokus_position-only"=1614807105, "set_x-Galvo_position-only_ticket"=1612714049, "set_y-Galvo_position-only_ticket"=1613762625, "set_z-Fokus_position-only_ticket"=1614811201, "read_x-Galvo_ticket"=1612714048, "read_y-Galvo_ticket"=1613762624, "read_z-Focus_ticket"=1614811200, "x-Galvo_pos_fromVar"=1612709955, "y-Galvo_pos_fromVar"=1613758531, "z-Focus_pos_fromVar"=1614807107] ("command")
  w61 = 10.0  # µs
  (unwired) u32 0 ("Delay 10µs")
  w82 = T4 4027518991 items=["read_x-Motor_status_ticket"=17305600, "init_x-Motor"=17760263, "read_x-Motor_absolute_ticket"=16781312, "move_x-Motor_absolute"=16777217, "move_x-Motor_relative"=16842753, "read_y-Motor_status_ticket"=18354176, "init_y-Motor"=18808839, "read_y-Motor_absolute_ticket"=17829888, "move_y-Motor_absolute"=17825793, "move_y-Motor_relative"=17891329, "read_z-Motor_status_ticket"=19402752, "init_z-Motor"=19857415, "stop_z-Motor"=19857423, "start_z-Motor"=19857422, "read_z-Motor_absolute_ticket"=18878464, "move_z-Motor_absolute"=18874369, "move_z-Motor_relative"=18939905, "end_no_ticket"=4027514895, "end_ticket"=4027518991, "IO-read_bank0"=3489665024, "IO-write_bank0"=3489660929, "IO-read_bank1"=3506442240, "IO-write_bank1"=3506438145, "IO-delay_bank0"=3489923073, "IO-delay_bank0_fromVar"=3489923075, "read_cam_clock"=3289124864, "store_cam_clock"=3289120770, "read_cam_phase"=3289190400, "set_cam_deadtime"=3288989697, "set_cam_10uscycles"=3289055233, "set_cam_10uscycles_fromVariable"=3289055235, "calc_cam"=3289317386, "store_cam_Var"=3289251842, "math_addToVariable"=4060086278, "readVar"=4060090368, "writeVar"=4060086273, "copyVar"=4060086276, "decrement_branchRel_if_equal"=4043374945, "decrement_branchRel_if_greaterequal"=4043375201, "decrement_branchRel_if_greaterequal_withTicket"=4043379297, "decrement_branchRel_if_smaller"=4043375457, "increment_branchRel_if_smaller"=4043375473, "set_x-Galvo"=1612710129, "set_y-Galvo"=1613758705, "set_z-Fokus"=1614807281, "set_x-Galvo_position-only"=1612709953, "set_y-Galvo_position-only"=1613758529, "set_z-Fokus_position-only"=1614807105, "set_x-Galvo_position-only_ticket"=1612714049, "set_y-Galvo_position-only_ticket"=1613762625, "set_z-Fokus_position-only_ticket"=1614811201, "read_x-Galvo_ticket"=1612714048, "read_y-Galvo_ticket"=1613762624, "read_z-Focus_ticket"=1614811200, "x-Galvo_pos_fromVar"=1612709955, "y-Galvo_pos_fromVar"=1613758531, "z-Focus_pos_fromVar"=1614807107] ("command")
  # "z-move"
  # "laser trig down"
  # "laser trig up"
  # "cam trig down"
  # "cam trig up"
  # "go back at end"
  n1 = Unbundle By Name("Constants") -> ("Camera-StartLine"=w27:u32, "Camera-Endline"=w28:u32, "zAccel"=w29:dbl, "SCMOS-LineSpeed [10µs]"=w26:dbl)  [unwired: 2 out]
  n2 = Unbundle By Name("User") -> ("z-distance_counts"=w3:i32, "#planes"=w2:u16, "exposue [10µs]"=w5:u32)
  n3 = Subtract(x=w28, y=w27) -> (x-y=w25:u32)
  n4 = Multiply(x=w25, y=w26) -> (x*y=w24:dbl)
  n5 = To Unsigned Long Integer(number=w24) -> (unsigned 32bit integer=w4:u32)
  "readout" <- w4
  n6 = call "MoveTime.vi"("maxaccel"=w29, "maxspeed"=w35, "dist"=w3) -> ()  [unwired: 1 out]
  n7 = Multiply(x=w3, y=w2) -> (x*y=w1:i32)
  n8 = Unbundle By Name("User") -> ("Digital-out"=w48:T9)
  n9 = Unbundle By Name("User") -> ("Digital-out"=w40:T9)
  n10 = call "SIAM-TMSI.vi"("Type"=enum8{"acc", "vel", "abs", "offset"}."offset", "Motor"=T8."z-Focus") -> ("Resolution-Factor"=w19:i32, "command"=w76:T4)  [unwired: 6 in, 2 out]
  n11 = Boolean To (0,1)(Boolean=TRUE) -> (0, 1=w50:i16)
  n12 = Boolean To (0,1)(Boolean=FALSE) -> (0, 1=w42:i16)
  n13 = To Unsigned Long Integer(number=w50) -> (unsigned 32bit integer=w49:u32)
  n14 = To Unsigned Long Integer(number=w42) -> (unsigned 32bit integer=w41:u32)
  n15 = Multiply(x=w19, y=w3) -> (x*y=w75:i32)
  n16 = Bundle By Name(cluster=w9, "Delay 10µs"=u32 0, "command"=w54, "P1"=w53) -> ()  [unwired: 1 out]
  n17 = To Long Integer(number=w75) -> (32bit integer=w20:i32)
  n18 = Logical Shift(y=w48, x=u32 1) -> (x << y=w47:u32)
  n19 = Logical Shift(y=w48, x=w49) -> (x << y=w46:u32)
  n20 = Logical Shift(y=w40, x=u32 1) -> (x << y=w39:u32)
  n21 = Logical Shift(y=w40, x=w41) -> (x << y=w38:u32)
  n22 = Bundle By Name(cluster=w9, "Delay 10µs"=u32 0, "command"=w52, "P0"=w47, "P1"=w46) -> (w33:T6)
  n23 = Bundle By Name(cluster=w9, "Delay 10µs"=w5, "command"=w76, "P0"=w20) -> (w22:T6)
  n24 = Bundle By Name(cluster=w9, "Delay 10µs"=u32 10, "command"=w59, "P0"=1, "P1"=1) -> (w32:T6)
  n25 = Bundle By Name(cluster=w9, "Delay 10µs"=u32 0, "command"=w17, "P0"=w15, "P1"=w2) -> (w8:T6)
  n26 = Bundle By Name(cluster=w9, "Delay 10µs"=u32 0, "command"=w44, "P0"=w39, "P1"=w38) -> (w21:T6)
  n27 = Bundle By Name(cluster=w9, "Delay 10µs"=u32 0, "command"=w14, "P0"=w10, "P1"=w13, "P2"=w11, "P5-ticket"=515) -> (w7:T6)
  n28 = Bundle By Name(cluster=w32, "Delay 10µs"=w4, "P1"=0) -> (w23:T6)
  n29 = Bundle By Name(cluster=w9, "Delay 10µs"=u32 10, "command"=w82, "P5-ticket"=112) -> (w80:T6)
  n30 = call "SIAM-TMSI.vi"("Type"=enum8{"acc", "vel", "abs", "offset"}."offset", "Motor"=T8."z-Focus") -> ("Resolution-Factor"=w71:i32, "command"=w72:T4)  [unwired: 6 in, 2 out]
  n31 = Negate(x=w1) -> (-x=w68:i32)
  n32 = Multiply(x=w71, y=w68) -> (x*y=w70:i32)
  n33 = Bundle By Name(cluster=w9, "Delay 10µs"=u32 50, "command"=w72, "P0"=w70) -> (w67:T6)
  n34 = Build Array(w33, w32, w8, w22, w7, w23, w21, w67, w80) -> (w60:T5)
  "SIAMScript" <- w60
  n35 = Multiply(x=w5, y=w61) -> (x*y=w62:dbl)
  n36 = Bundle By Name(cluster=T7 {"Camera-Exposure"=550.5, "CameraImages"=245} ("Cluster"), "Camera-Exposure"=w62, "CameraImages"=w2) -> (→"Camera":T7)
  n37 = Array Size(array=w60) -> (size(s)=→"size(s)":i32)
  "error out" <- "error in (no error)"
